vi "Close Hardware.vi"(8 "error in (no error)":errorcluster, 11 "Inst.TC in":refnum<class "Inst.TC.lvclass">) -> (0 "error out":errorcluster, 3 "Inst.TC out":refnum<class "Inst.TC.lvclass">)   [LabVIEW 2019, in "Inst.TC.lvclass"]
uses:
  Inst.TC.lvclass
  <userlib>/LevyLab/Instrument Framework/Instrument Types/VSource/Instrument.VSource.lvclass
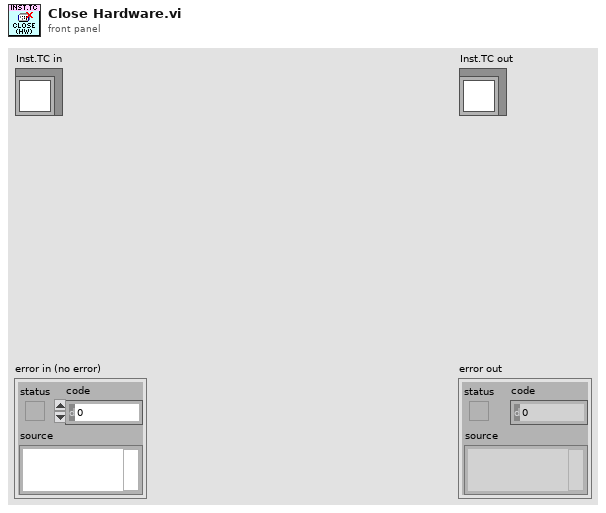
[diagram p1: front panel]
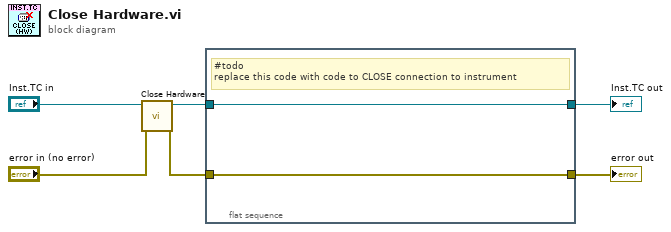
[diagram p0: block diagram]
diagram:
  n1 = call-parent "Close Hardware.vi"("error in (no error)"="error in (no error)", "Instrument in"="Inst.TC in") -> ("error out"=w4:errorcluster, "Instrument out"=w2:refnum<class "Inst.TC.lvclass">)  [unwired: 8 in]
  n2 = flat-sequence {
    tunnel: w4 -> [w8]
    tunnel: [w8] -> w3
    tunnel: w2 -> [w7]
    tunnel: [w7] -> w1
    frame #0 {
      # "#todo\nreplace this code with code to CLOSE connection to instrument"
    }
  }
  "error out" <- w3
  "Inst.TC out" <- w1
